vi "Prepare Device.vi"(2 "error in (no error)":errorcluster, 3 "SPI Device":T2) -> (1 "SPI Device":T2)   [LabVIEW 2010]
uses:
  Controls/SpiDevice.ctl
panel:
  out "High IO Values":T1
  out "Result":u32
  out "error out":errorcluster
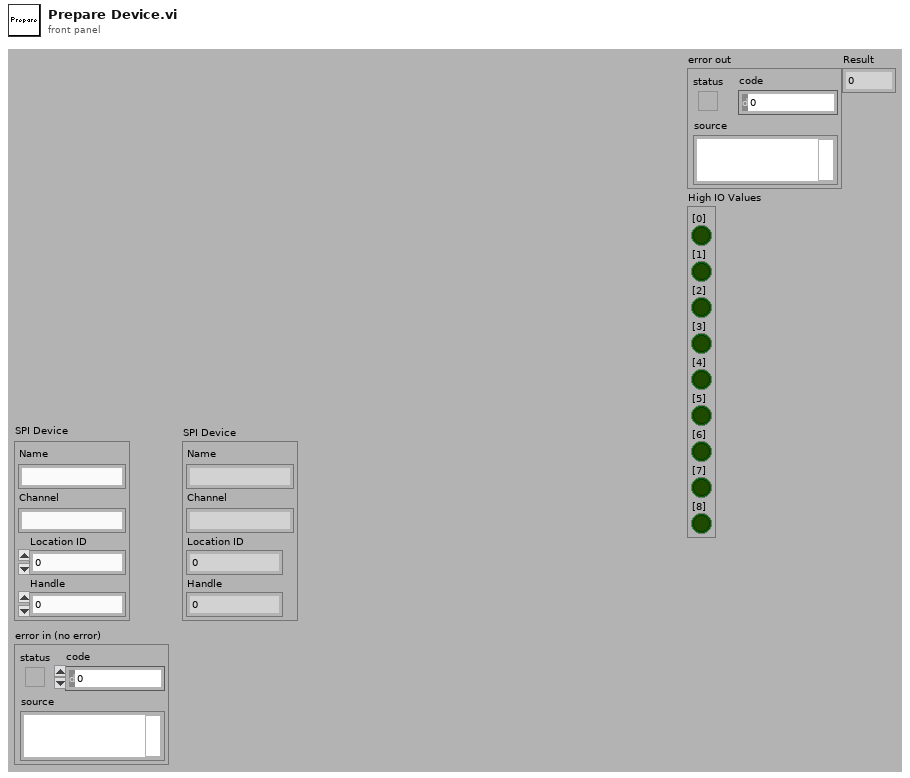
[diagram p1: front panel]
types:
  T1 = cluster{"[0]":bool, "[1]":bool, "[2]":bool, "[3]":bool, "[4]":bool, "[5]":bool, "[6]":bool, "[7]":bool, "[8]":bool}
  T2 = typedef "SpiDevice.ctl" = cluster{"Name":string, "Channel":string, "Location ID":u32, "Handle":u32}
  T3 = cluster{"ADBUS3 Chip Select":bool, "ADBUS4 GPIO1L":bool, "ADBUS5 GPIO1L":bool, "ADBUS6 GPIO1L":bool, "ADBUS7 GPIO1L":bool}
  T4 = cluster{"Pin 1 I/O":bool, "Pin 1 L/H":bool, "Pin 2 I/O":bool, "Pin 2 L/H":bool, "Pin 3 I/O":bool, "Pin 3 L/H":bool, "Pin 4 I/O 2":bool, "Pin 4 L/H":bool, "Pin 5 I/O":bool, "Pin 5 L/H":bool, "Pin 6 I/O":bool, "Pin 6 L/H":bool, "Pin 7 I/O":bool, "Pin 7 L/H":bool, "Pin 8 I/O":bool, "Pin 8 L/H":bool}
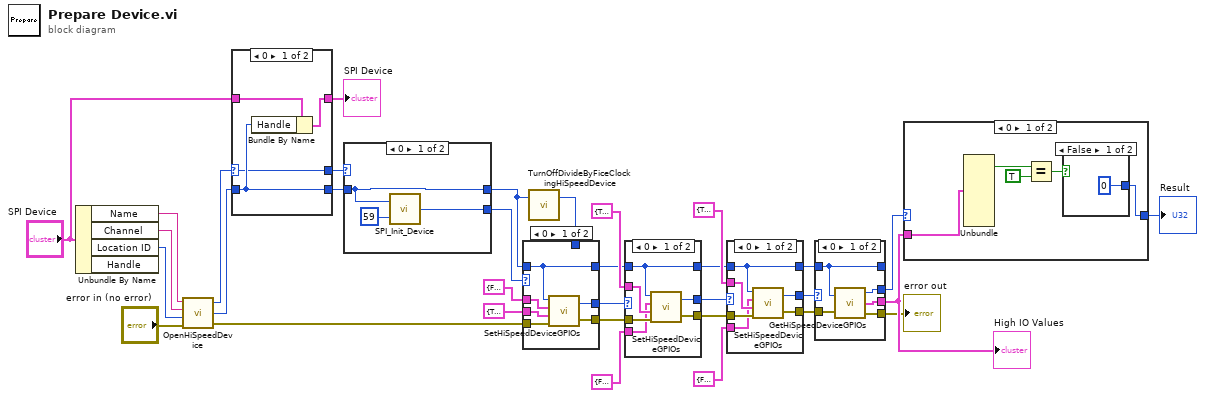
[diagram p0: block diagram]
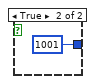
[diagram p2: hidden frame]
diagram:
  n1 = Unbundle By Name("SPI Device") -> ("Name"=w33:string, "Channel"=w32:string, "Location ID"=w31:u32)  [unwired: 1 out]
  n2 = call "OpenHiSpeedDevice.vi"("error in (no error)"="error in (no error)", "Location ID"=w31, "Device channel"=w32, "Device name"=w33) -> ("error out"=w22:errorcluster, "Handle"=w27:u32, "Result"=w28:u32)
  n3 = case shown="0" w28 {
    selector: w28 -> [w34 w38]
    tunnel: "SPI Device" -> [w37 w40]
    tunnel: w27 -> [w35 w39]
    tunnel: [w36 w40] -> w26
    tunnel: [w35 w39] -> w24
    tunnel: [w34 w38] -> w25
    frame 0 {
      n4 = Bundle By Name(cluster=w37, "Handle"=w35) -> (w36:T2)
    }
    frame Default {
    }
  }
  "SPI Device" <- w26
  n5 = case shown="0" w25 {
    selector: w25 -> [_ w45]
    tunnel: [w43 w45] -> w23
    tunnel: w24 -> [w41 w44]
    tunnel: [w41 w44] -> w2
    frame 0 {
      n6 = call "SPI_Init_Device.vi"("ClockDivisor"=u32 59, "Handle"=w41) -> ("FTC_Status"=w43:u32)
    }
    frame Default {
    }
  }
  n7 = call "TurnOffDivideByFiceClockingHiSpeedDevice.vi"("handle"=w2) -> ("result"=w1:u32)  [unwired: 1 in, 1 out]
  n8 = case shown="0" w23 {
    selector: w23 -> [_ w53]
    tunnel: w2 -> [w50 w54]
    tunnel: [w50 w54] -> w17
    tunnel: [w51 w53] -> w16
    tunnel: w22 -> [w49 w52]
    tunnel: T4 {"Pin 1 I/O"=TRUE, "Pin 1 L/H"=TRUE, "Pin 2 I/O"=FALSE, "Pin 2 L/H"=FALSE, "Pin 3 I/O"=FALSE, "Pin 3 L/H"=FALSE, "Pin 4 I/O 2"=FALSE, "Pin 4 L/H"=FALSE, "Pin 5 I/O"=FALSE, "Pin 5 L/H"=FALSE, "Pin 6 I/O"=FALSE, "Pin 6 L/H"=FALSE, "Pin 7 I/O"=FALSE, "Pin 7 L/H"=FALSE, "Pin 8 I/O"=FALSE, "Pin 8 L/H"=FALSE} ("Input Output Pins") -> [w48 _]
    tunnel: T3 {"ADBUS3 Chip Select"=FALSE, "ADBUS4 GPIO1L"=FALSE, "ADBUS5 GPIO1L"=FALSE, "ADBUS6 GPIO1L"=FALSE, "ADBUS7 GPIO1L"=FALSE} ("Chip Select Disable States") -> [w47 _]
    tunnel: [w46 w52] -> w15
    tunnel: w1 -> [_ _]
    frame 0 {
      n9 = call "SetHiSpeedDeviceGPIOs.vi"("error in (no error)"=w49, "Input Output Pins"=w48, "Chip Select Disable States"=w47, "Handle"=w50) -> ("error out"=w46:errorcluster, "Result"=w51:u32)
    }
    frame Default {
    }
  }
  n10 = case shown="0" w16 {
    selector: w16 -> [_ w62]
    tunnel: w17 -> [w59 w63]
    tunnel: [w59 w63] -> w12
    tunnel: [w60 w62] -> w11
    tunnel: w15 -> [w58 w61]
    tunnel: T4 {"Pin 1 I/O"=TRUE, "Pin 1 L/H"=FALSE, "Pin 2 I/O"=FALSE, "Pin 2 L/H"=FALSE, "Pin 3 I/O"=FALSE, "Pin 3 L/H"=FALSE, "Pin 4 I/O 2"=FALSE, "Pin 4 L/H"=FALSE, "Pin 5 I/O"=FALSE, "Pin 5 L/H"=FALSE, "Pin 6 I/O"=FALSE, "Pin 6 L/H"=FALSE, "Pin 7 I/O"=FALSE, "Pin 7 L/H"=FALSE, "Pin 8 I/O"=FALSE, "Pin 8 L/H"=FALSE} ("Input Output Pins") -> [w57 _]
    tunnel: T3 {"ADBUS3 Chip Select"=FALSE, "ADBUS4 GPIO1L"=FALSE, "ADBUS5 GPIO1L"=FALSE, "ADBUS6 GPIO1L"=FALSE, "ADBUS7 GPIO1L"=FALSE} ("Chip Select Disable States") -> [w56 _]
    tunnel: [w55 w61] -> w10
    frame 0 {
      n11 = call "SetHiSpeedDeviceGPIOs.vi"("error in (no error)"=w58, "Input Output Pins"=w57, "Chip Select Disable States"=w56, "Handle"=w59) -> ("error out"=w55:errorcluster, "Result"=w60:u32)
    }
    frame Default {
    }
  }
  n12 = case shown="0" w11 {
    selector: w11 -> [_ w71]
    tunnel: w12 -> [w68 w72]
    tunnel: [w68 w72] -> w7
    tunnel: [w69 w71] -> w9
    tunnel: w10 -> [w67 w70]
    tunnel: T4 {"Pin 1 I/O"=TRUE, "Pin 1 L/H"=TRUE, "Pin 2 I/O"=FALSE, "Pin 2 L/H"=FALSE, "Pin 3 I/O"=FALSE, "Pin 3 L/H"=FALSE, "Pin 4 I/O 2"=FALSE, "Pin 4 L/H"=FALSE, "Pin 5 I/O"=FALSE, "Pin 5 L/H"=FALSE, "Pin 6 I/O"=FALSE, "Pin 6 L/H"=FALSE, "Pin 7 I/O"=FALSE, "Pin 7 L/H"=FALSE, "Pin 8 I/O"=FALSE, "Pin 8 L/H"=FALSE} ("Input Output Pins") -> [w66 _]
    tunnel: T3 {"ADBUS3 Chip Select"=FALSE, "ADBUS4 GPIO1L"=FALSE, "ADBUS5 GPIO1L"=FALSE, "ADBUS6 GPIO1L"=FALSE, "ADBUS7 GPIO1L"=FALSE} ("Chip Select Disable States") -> [w65 _]
    tunnel: [w64 w70] -> w8
    frame 0 {
      n13 = call "SetHiSpeedDeviceGPIOs.vi"("error in (no error)"=w67, "Input Output Pins"=w66, "Chip Select Disable States"=w65, "Handle"=w68) -> ("error out"=w64:errorcluster, "Result"=w69:u32)
    }
    frame Default {
    }
  }
  n14 = case shown="0" w9 {
    selector: w9 -> [_ w79]
    tunnel: w8 -> [w77 w78]
    tunnel: w7 -> [w76 w80]
    tunnel: [w76 w80] -> _
    tunnel: [w75 w79] -> w6
    tunnel: [w74 _] -> w5
    tunnel: [w73 w78] -> w4
    frame 0 {
      n15 = call "GetHiSpeedDeviceGPIOs.vi"("Handle"=w76, "error in (no error)"=w77) -> ("Result"=w75:u32, "High IO Values"=w74:T1, "error out"=w73:errorcluster)
    }
    frame Default {
    }
  }
  "error out" <- w4
  "High IO Values" <- w5
  n16 = case shown="0" w6 {
    selector: w6 -> [_ w88]
    tunnel: w5 -> [w85 _]
    tunnel: [w81 w88] -> w3
    frame 0 {
      n17 = Unbundle(w85) -> ("[1]"=w84:bool)  [unwired: 8 out]
      n18 = Equal?(x=w84, y=TRUE) -> (x = y?=w82:bool)
      n19 = case shown="False" w82 {
        tunnel: [u32 0 u32 1001] -> w81
        frame False {
        }
        frame True {
        }
      }
    }
    frame Default {
    }
  }
  "Result" <- w3
